vi "MCP4725 Generate and Read Example 3.vi"(8 "Error In":errorcluster) -> (0 "Error Out":errorcluster)   [LabVIEW 2014]
doc: "This example produces stepped triangle wave on output in loop, there's no timing inside while loop so it's running as fast as it can, at test computer signal has frequency 440Hz and consists from 12 samples, so we are able to produce this fast signals at most."
uses:
  LabVIEW-Universal-Transcriptor-MCP4725/MCP4725.lvclass
  <vilib>/LabVIEW Universal Transcriptor/LabVIEW to Arduino Transcriptor/Transcriptors/System API/Serial println string.vi
panel:
  # "This example produces stepped triangle wave on output in loop, there's no timing inside while loop so it's running as fast as it can, at test computer signal has frequency 440Hz and consists from 12 samples, so we are able to produce this fast signals at most.\n\nWiring:\n  Arduino Nano  |  MCP4725 module\n  -----------------------------------------\n          VCC        |           +5V\n          GND        |           GND\n          A4           |           SDA\n          A5           |           SCL"
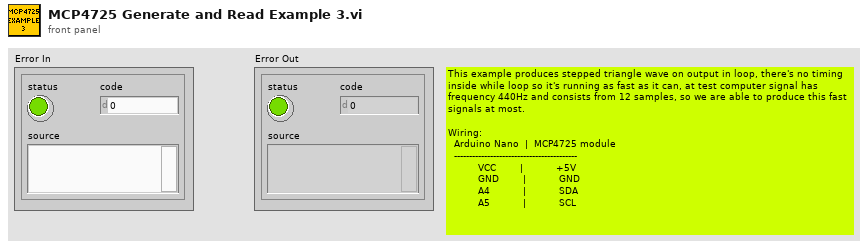
[diagram p1: front panel]
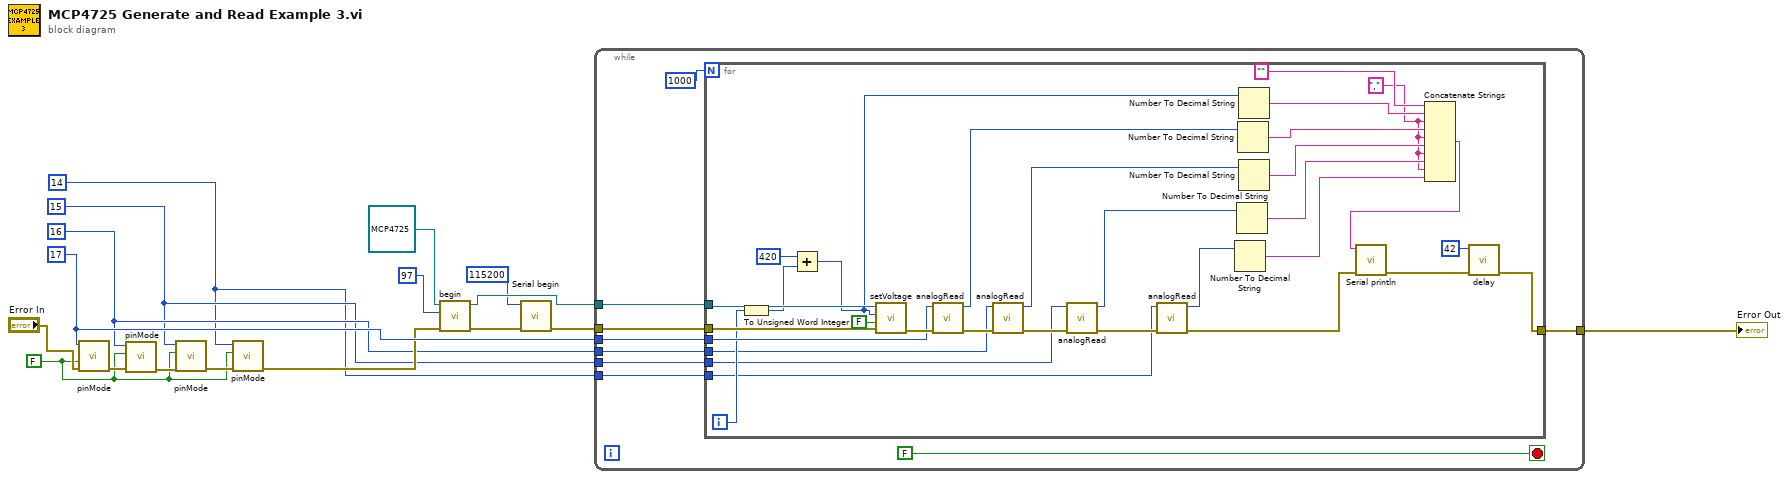
[diagram p0: block diagram]
diagram:
  w1 = 14 ("pin number")
  w2 = 15 ("pin number")
  w3 = 16 ("pin number")
  w5 = FALSE ("output?")
  w12 = 17 ("pin number")
  n1 = call <vilib>:"pinMode.vi"("Error In"="Error In", "output?"=w5, "pin number"=w12) -> ("Error Out"=w8:errorcluster)  [unwired: 8 in]
  n2 = call <vilib>:"pinMode.vi"("Error In"=w8, "output?"=w5, "pin number"=w3) -> ("Error Out"=w7:errorcluster)  [unwired: 8 in]
  n3 = call <vilib>:"pinMode.vi"("Error In"=w7, "output?"=w5, "pin number"=w2) -> ("Error Out"=w6:errorcluster)  [unwired: 8 in]
  n4 = call <vilib>:"pinMode.vi"("Error In"=w6, "output?"=w5, "pin number"=w1) -> ("Error Out"=w4:errorcluster)  [unwired: 8 in]
  n5 = call "begin.vi"("error in (no error)"=w4, "I2C addr"=u8 97, "MCP4725 in"=refnum<class "MCP4725.lvclass"> refnum) -> ("error out"=w11:errorcluster, "MCP4725 out"=w16:refnum<class "MCP4725.lvclass">)  [unwired: 7 in]
  n6 = call <vilib>:"Serial begin.vi"("Error In"=w11, "speed (Bd)"=115200) -> ("Error Out"=w10:errorcluster)  [unwired: 9 in]
  n7 = while {
    tunnel: w10 -> [w25]
    tunnel: w16 -> [w24]
    tunnel: [w23] -> w15
    tunnel: w12 -> [w22]
    tunnel: w3 -> [w20]
    tunnel: w2 -> [w19]
    tunnel: w1 -> [w18]
    stop <- FALSE stop-if-true
    n8 = for {
      N: 1000 -> [_]
      tunnel: w25 -> [w57]
      tunnel: w24 -> [w56]
      tunnel: [w46] -> w23
      tunnel: w22 -> [w53]
      tunnel: w20 -> [w36]
      tunnel: w19 -> [w35]
      tunnel: w18 -> [w34]
      i -> [w48]
      w27 = "," ("string")
      n9 = To Unsigned Word Integer(number=w48) -> (unsigned 16bit integer=w43:u16)
      n10 = Add(x=u16 420, y=w43) -> (x+y=w42:u16)
      n11 = call "setVoltage.vi"("error in (no error)"=w57, "writeEEPROM?"=FALSE, "voltage"=w42, "MCP4725 in"=w56) -> ("error out"=w54:errorcluster)  [unwired: 6 in, 1 out]
      n12 = call <vilib>:"analogRead.vi"("Error In"=w54, "pin number"=w53) -> ("Error Out"=w41:errorcluster, "value"=w40:u16)  [unwired: 8 in]
      n13 = call <vilib>:"analogRead.vi"("Error In"=w41, "pin number"=w36) -> ("Error Out"=w39:errorcluster, "value"=w33:u16)  [unwired: 8 in]
      n14 = call <vilib>:"analogRead.vi"("Error In"=w39, "pin number"=w35) -> ("Error Out"=w38:errorcluster, "value"=w32:u16)  [unwired: 8 in]
      n15 = call <vilib>:"analogRead.vi"("Error In"=w38, "pin number"=w34) -> ("Error Out"=w37:errorcluster, "value"=w31:u16)  [unwired: 8 in]
      n16 = Number To Decimal String(number=w31) -> (decimal integer string=w28:string)  [unwired: 1 in]
      n17 = Number To Decimal String(number=w32) -> (decimal integer string=w29:string)  [unwired: 1 in]
      n18 = Number To Decimal String(number=w40) -> (decimal integer string=w50:string)  [unwired: 1 in]
      n19 = Number To Decimal String(number=w42) -> (decimal integer string=w52:string)  [unwired: 1 in]
      n20 = Number To Decimal String(number=w33) -> (decimal integer string=w30:string)  [unwired: 1 in]
      n21 = Concatenate Strings("" ("string"), w52, w27, w50, w27, w30, w27, w29, w27, w28) -> (w49:string)
      n22 = call-poly <vilib>:"Serial println.vi"("Error In"=w37, "string in"=w49) -> ("Error Out"=w47:errorcluster)  [unwired: 9 in]
      n23 = call <vilib>:"delay.vi"("Error In"=w47, "time (ms)"=42) -> ("Error Out"=w46:errorcluster)  [unwired: 9 in]
    }
  }
  "Error Out" <- w15
